vi "IntakeOutput.vi"   [LabVIEW 2017]
uses:
  IntakeOutput.ctl
  <vilib>/Rock Robotics/WPI/ThirdParty/Phoenix-LabVIEW/Motor Controller/Controls/CTRE_Phoenix_MotorControl_ControlMode.ctl
types:
  T1 = typedef "IntakeOutput.ctl" = cluster{"Control Mode":T2, "LeftIntakeSetting":dbl, "RightIntakeSetting":dbl}
  T2 = typedef "CTRE_Phoenix_MotorControl_ControlMode.ctl" = u16
  T3 = typedef "WPI_MotorControlDeviceRef.ctl" = cluster{"DeviceStatus":errorcluster, "Type":T4, "PWM":cluster{"PWM Channel":T5, "DeadBand":T6}, "CAN":cluster{"Device Number":u8, "SetOutput VI Ref":variant, "GetOutput VI Ref":variant, "Enable VI Ref":variant, "Disable VI Ref":variant, "Data":variant}, "Invert":bool, "DIO PWM":cluster{"PWM \"Enable\" Channel":T5, "DIOChannel":T7, "PWM Rate":dbl}}
  T4 = typedef "WPI_MotorControlType.ctl" = enum16{"PWM", "CAN", "DIO PWM"}
  T5 = typedef "FPGA_DIOPWMChannel.ctl" = enum8{"PWM 0", "PWM 1", "PWM 2", "PWM 3", "PWM 4", "PWM 5", "PWM 6", "PWM 7", "PWM 8", "PWM 9", "PWM MXP 0", "PWM MXP 1", "PWM MXP 2", "PWM MXP 3", "PWM MXP 4", "PWM MXP 5", "PWM MXP 6", "PWM MXP 7", "PWM MXP 8", "PWM MXP 9", "Invalid"}
  T6 = typedef "WPI_PWMDeadband.ctl" = cluster{"Name":string, "maxPositivePwm":i32, "minPositivePwm":i32, "centerPwm":i32, "maxNegativePwm":i32, "minNegativePwm":i32, "angularRange":u16}
  T7 = typedef "FPGA_DIOChannel.ctl" = enum8{"DIO 0", "DIO 1", "DIO 2", "DIO 3", "DIO 4", "DIO 5", "DIO 6", "DIO 7", "DIO 8", "DIO 9", "DIO MXP 0", "DIO MXP 1", "DIO MXP 2", "DIO MXP 3", "DIO MXP 4", "DIO MXP 5", "DIO MXP 6", "DIO MXP 7", "DIO MXP 8", "DIO MXP 9", "DIO MXP 10", "DIO MXP 11", "DIO MXP 12", "DIO MXP 13", "DIO MXP 14", "DIO MXP 15", "SPI Port CS1", "SPI Port CS2", "SPI Port CS3", "SPI Port MISO", "SPI Port MOSI", "Invalid"}
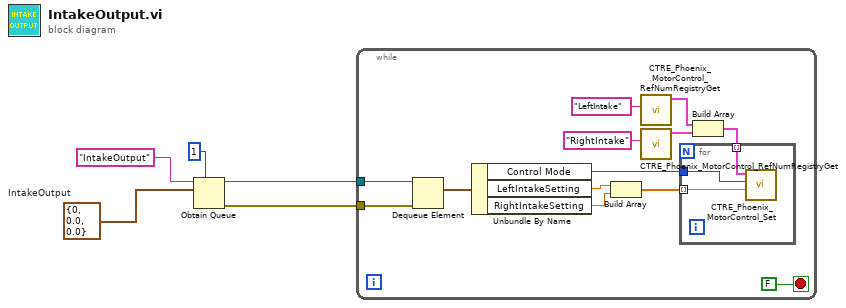
[diagram p0: block diagram]
diagram:
  w4 = T1 {"Control Mode"=0, "LeftIntakeSetting"=0.0, "RightIntakeSetting"=0.0}  # IntakeOutput
  n1 = Obtain Queue(max queue size (-1, unlimited)=1, name (unnamed)="IntakeOutput", element data type=w4) -> (queue out=w3:refnum<queue>, error out=w2:errorcluster)  [unwired: 2 in, 1 out]
  n2 = while {
    tunnel: w3 -> [w12]
    tunnel: w2 -> [w11]
    stop <- FALSE stop-if-true
    n3 = Dequeue Element(queue=w12, error in (no error)=w11) -> (element=w10:T1)  [unwired: 1 in, 3 out]
    n4 = Unbundle By Name(w10) -> ("Control Mode"=w6:T2, "LeftIntakeSetting"=w8:dbl, "RightIntakeSetting"=w7:dbl)
    n5 = Build Array(w8, w7) -> (w13:dbl[])
    n6 = call <vilib>:"CTRE_Phoenix_MotorControl_RefNumRegistryGet.vi"("refnum name"="LeftIntake") -> ("PhoenixMotorControlDevRef"=w18:T3)  [unwired: 9 in, 1 out]
    n7 = call <vilib>:"CTRE_Phoenix_MotorControl_RefNumRegistryGet.vi"("refnum name"="RightIntake") -> ("PhoenixMotorControlDevRef"=w17:T3)  [unwired: 9 in, 1 out]
    n8 = Build Array(w18, w17) -> (w16:T3[])
    n9 = for {
      tunnel: w6 -> [w21]
      tunnel: w16 -> [w20] mode=indexing
      tunnel: w13 -> [w19] mode=indexing
      n10 = call <vilib>:"CTRE_Phoenix_MotorControl_Set.vi"("Output"=w19, "Control Mode"=w21, "PhoenixMotorControlDevRef"=w20) -> ()  [unwired: 7 in, 2 out]
    }
  }
